vi "filtring.vi"() -> ()   [LabVIEW 2020]
uses:
  <vilib>/Analysis/5stat.llb/RMS (DBL).vi
  <vilib>/measure/matone.llb/Extract Multiple Tone Information 1 Chan.vi
  <vilib>/express/express analysis/Spectral/Block/exnSpectralBlock spectral measurements RMS poly.vi
  <vilib>/express/express analysis/Spectral/Block/exnSpectralBlock spectral measurements RMS WFM.vi
  <vilib>/express/express analysis/Spectral/Block/exnSpectralBlock spectral measurements RMS DDT.vi
  <vilib>/express/express analysis/Spectral/XNode/ExpressSpectralMeasurementsBlockNode.xnode
  <vilib>/measure/NI_MABase.lvlib
  <vilib>/Analysis/NI_AALPro.lvlib
  <vilib>/measure/NI_MAPro.lvlib
panel:
  in  "threshold 2":dbl=0.001 format="%#_6p"
  out "multiple tone information filtred":T1(array[cluster]) {"detected phase (deg)" format="%_6g"; "detected amplitude" format="%_6p"; "detected frequency" format="%_6p"}
  out "multiple tone information":T1(array[cluster]) {"detected phase (deg)" format="%_6g"; "detected amplitude" format="%_6p"; "detected frequency" format="%_6p"}
  in  "threshold":dbl=0.001 format="%#_6p"
  out "rms value filtred":dbl format="%0.2f"
  out "rms value":dbl format="%0.2f"
  out "fft filtred":dynamicdata(graph)
  out "fft":cluster{"f0":dbl, "df":dbl, "magnitude":dbl[]}(graph)
  out "filtred":dynamicdata(graph)
  out "squre wave":waveform(dbl)(graph)
  in  "Knob":dbl(knob) scale=0.0..500.0
  in  "signal type":T2(ring)
  in  "N":dbl=10.0 format="%0.2p"
  in  "fs":dbl=1.0 format="%0.2p"
  in  "frequency":dbl=10.0 format="%0.2p"
  in  "amplitude":dbl=1.0 format="%0.2p"
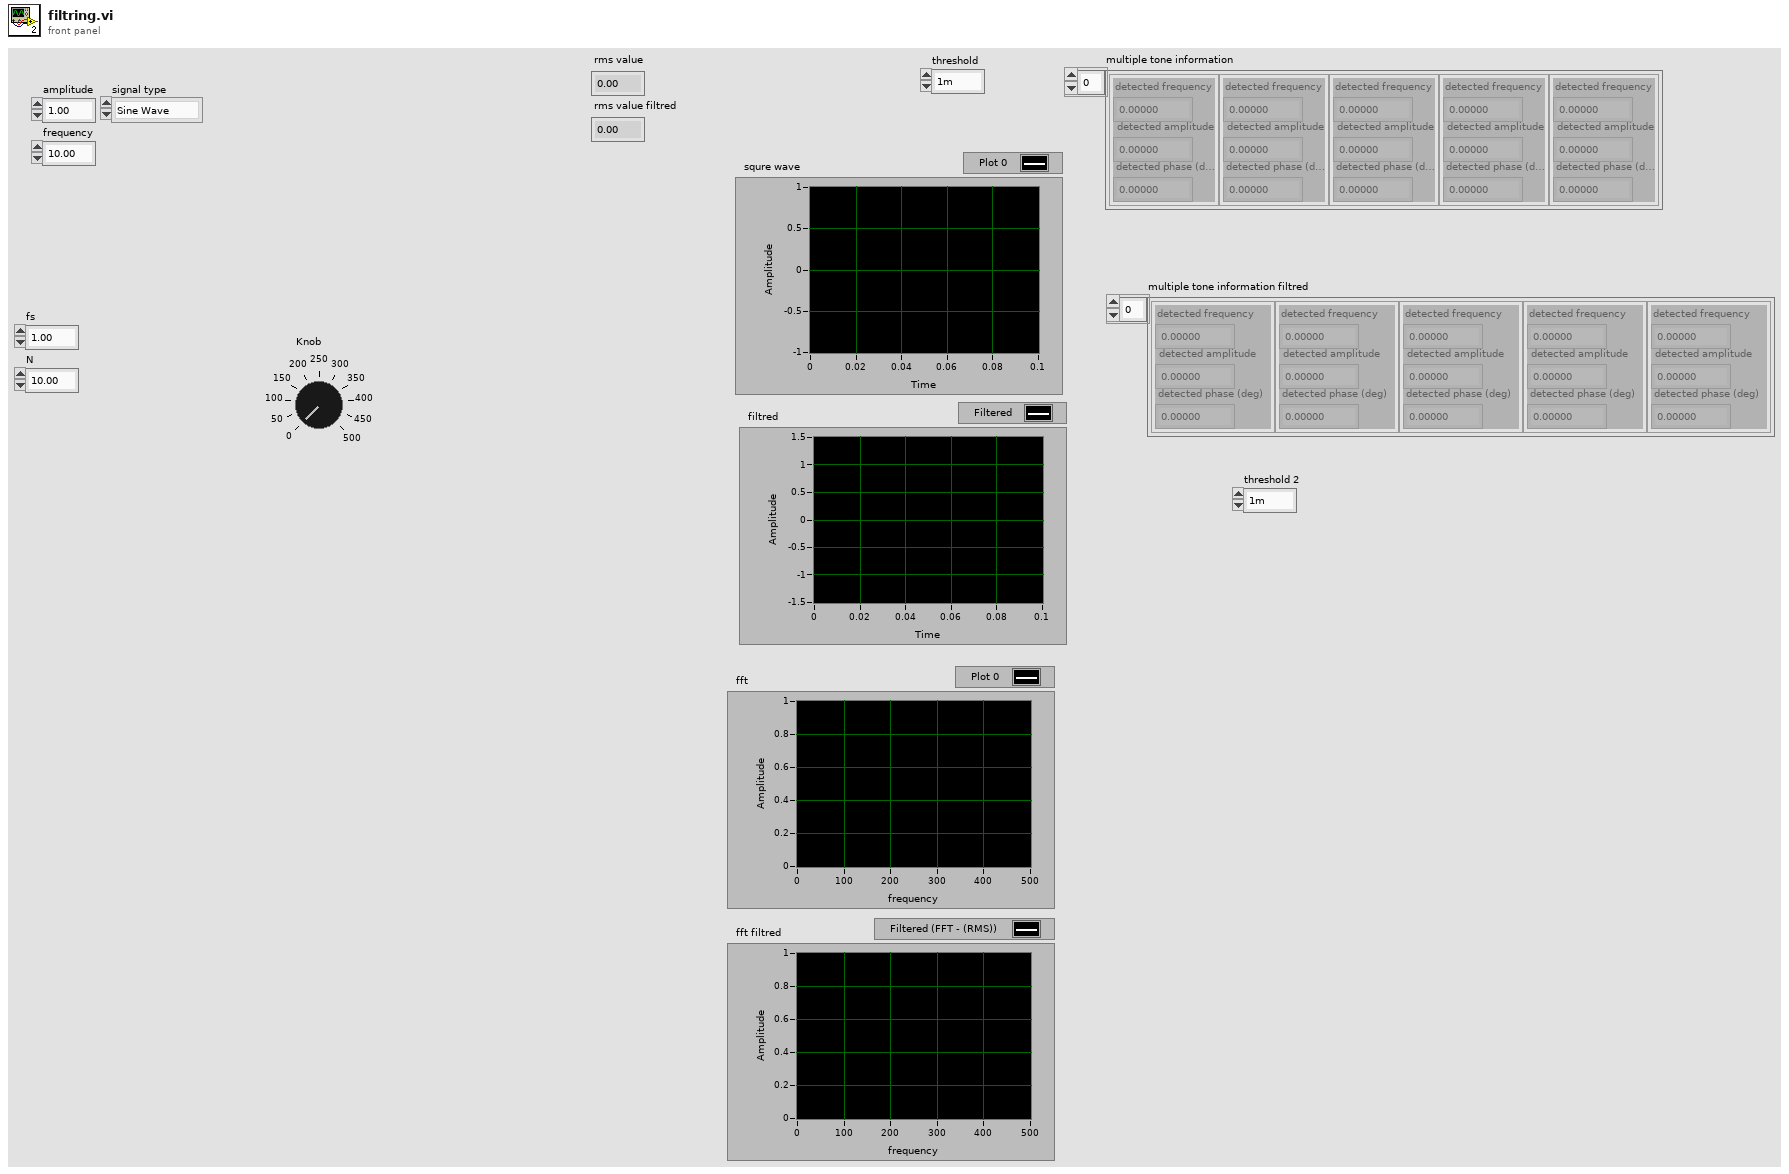
[diagram p1: front panel]
types:
  T1 = cluster{"detected frequency":dbl, "detected amplitude":dbl, "detected phase (deg)":dbl}[]
  T2 = enum16{"Sine Wave", "Triangle Wave", "Square Wave", "Sawtooth Wave"}
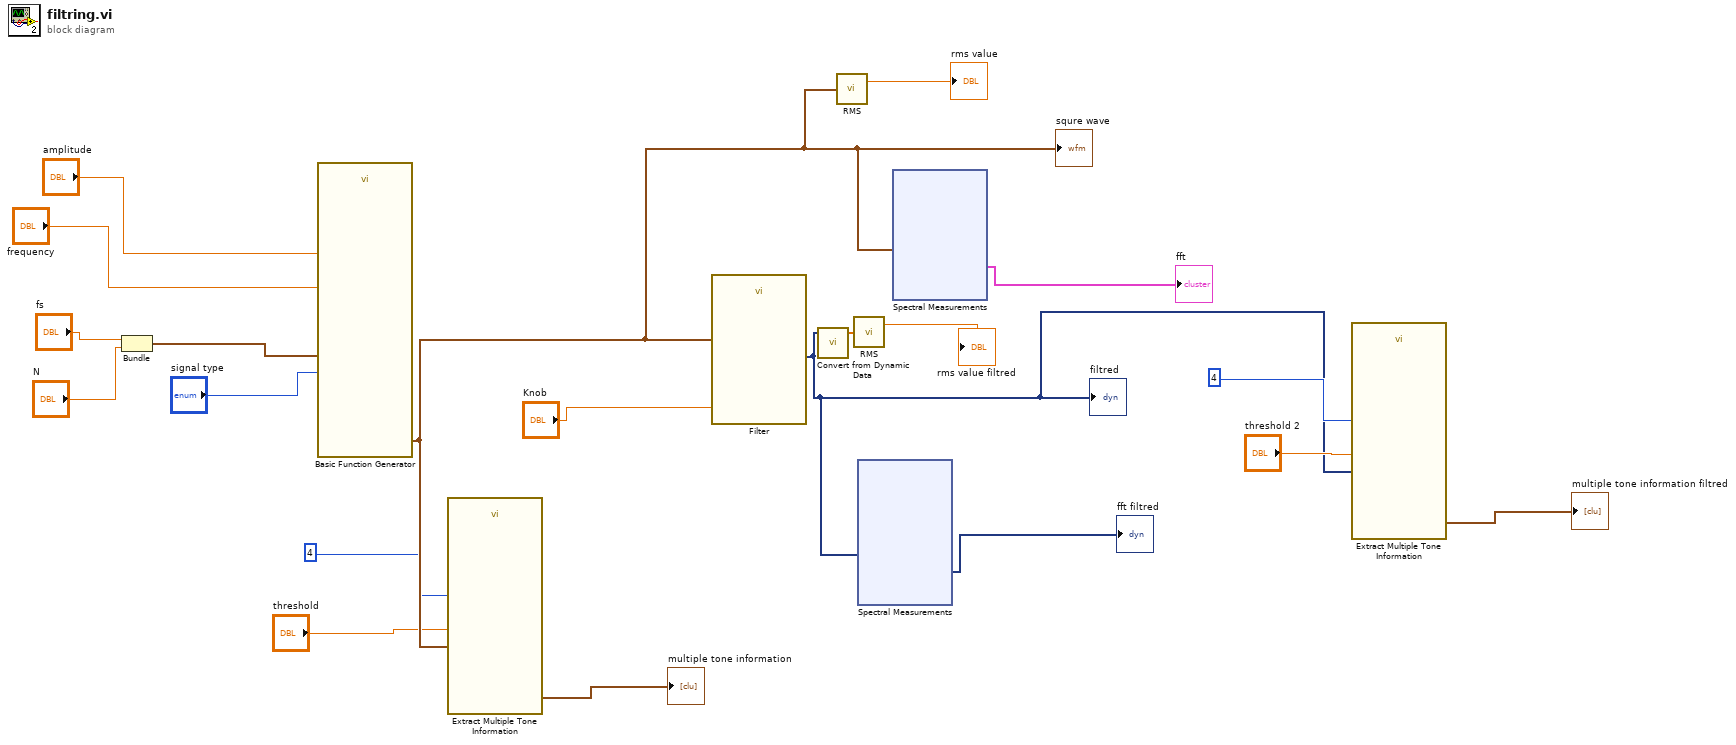
[diagram p0: block diagram]
diagram:
  n1 = Bundle("fs"="fs", "N"="N") -> (w16:cluster{"fs":dbl, "N":dbl})  [unwired: 1 in]
  n2 = call <vilib>:"Basic Function Generator.vi"("sampling info"=w16, "signal type"="signal type", "amplitude"="amplitude", "frequency"="frequency") -> ("signal out"=w8:waveform(dbl))  [unwired: 5 in, 2 out]
  "squre wave" <- w8
  n3 = call-poly <vilib>:"Extract Multiple Tone Information.vi"("time signal in"=w8, "threshold"="threshold", "max num tones"=4) -> ("multiple tone information"=→"multiple tone information":T1)  [unwired: 10 in, 2 out]
  n4 = call "Filter"("Lower Cut-Off"="Knob", "Signal"=w8) -> ("Filtered Signal"=w1:dynamicdata)  [unwired: 8 in, 1 out]
  "filtred" <- w1
  n5 = call "Convert from Dynamic Data"("Dynamic Data Type"=w1) -> ("Array"=w11:dbl[])  [unwired: 3 in]
  n6 = call-poly <vilib>:"RMS.vi"("X"=w8) -> ("rms value"=→"rms value":dbl)  [unwired: 1 out]
  n7 = call-poly <vilib>:"RMS.vi"("X"=w11) -> ("rms value"=→"rms value filtred":dbl)  [unwired: 1 out]
  n8 = xnode "Spectral Measurements"("Signals"=w1) -> ("FFT - (RMS)"=→"fft filtred":dynamicdata)  [unwired: 1 in, 2 out]
  n9 = xnode "Spectral Measurements"("Signals"=w8) -> ("FFT - (RMS)"=→"fft":cluster{"f0":dbl, "df":dbl, "magnitude":dbl[]})  [unwired: 1 in, 2 out]
  n10 = call-poly <vilib>:"Extract Multiple Tone Information.vi"("time signal in"=w1, "threshold"="threshold 2", "max num tones"=4) -> ("multiple tone information"=→"multiple tone information filtred":T1)  [unwired: 10 in, 2 out]
